vi "CRYDB Insert Into DatarunTable.vi"(6 "Station_ID":i32, 7 "Item_ID":i32, 8 "error in":errorcluster, 10 "Auto save":T1 {"Selector" items=["Space", "Underscores", "None"]}, 11 "connection reference":T2) -> (0 "error out":errorcluster, 2 "Datarun_ID":i32, 3 "connection reference out":T2)   [LabVIEW 2013]
uses:
  <vilib>/addons/database/Connection.llb/Conn ObjectReference.ctl
  Typedef Control/CRYAuto Save Cluster.ctl
  <vilib>/addons/database/Auxilliary.llb/DB Tools Column Info.ctl
  <vilib>/addons/database/Auxilliary.llb/DB Tools DataTypes.ctl
  Calibration/SubVI/CRYCal Global.vi
  CRYProject/CRYProject Editor Global.vi
  <vilib>/addons/database/Connection.llb/Conn Execute.vi
  <vilib>/addons/database/Recordset.llb/Rec Fetch Recordset Data (R).vi
  <vilib>/addons/database/Recordset.llb/Rec Destroy - Connection.vi
  <vilib>/addons/database/_DB Variant To Data/Database Variant To Data.xnode
  <vilib>/addons/database/NI_Database_API.lvlib
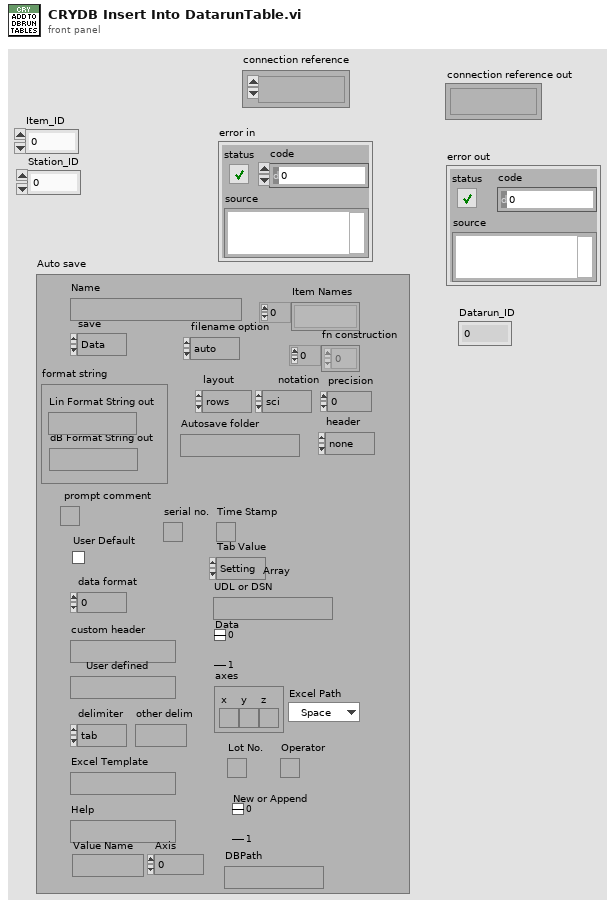
[diagram p1: front panel]
types:
  T1 = typedef "CRYAuto Save Cluster.ctl" = cluster{"Name":string, "save":enum16{"Data", "Results", "Waveforms"}, "Item Names":string[], "Autosave folder":path, "data format":u16, "filename option":enum16{"auto", "prompt"}, "fn construction":i32[], "layout":enum16{"rows", "columns"}, "notation":enum16{"sci", "float"}, "precision":i32, "prompt comment":bool, "header":enum16{"none", "standard", "custom"}, "custom header":string, "serial no.":bool, "User defined":string, "delimiter":enum16{"tab", "comma", "space", "other"}, "other delim":string, "axes":cluster{"x":bool, "y":bool, "z":bool}, "Time Stamp":bool, "Lot No.":bool, "Operator":bool, "Excel Template":string, "New or Append":u16, "Data":u16, "Help":string, "Tab Value":enum32{"Setting", "Help"}, "UDL or DSN":path, "User Default":bool, "Selector":i32, "Axis":u16, "Value Name":string, "format string":cluster{"dB Format String out":string, "Lin Format String out":string}, "DBPath":path}
  T2 = typedef "NI_Database_API.lvlib/Conn ObjectReference.ctl" = refnum<k1>
  T3 = typedef "NI_Database_API.lvlib/DB Tools Column Info.ctl" = cluster{"column name":string, "data type":T4, "size":i32, "allow null?":bool}
  T4 = typedef "NI_Database_API.lvlib/DB Tools DataTypes.ctl" = enum16{"String", "Long (I32)", "Single (SGL)", "Double (DBL)", "Date/Time", "Binary"}
  T5 = cluster{"Datarun_ID":u32, "Station_ID":i32, "Operator":string, "TStamp":string, "Item_ID":i32, "Comment":string, "Seq Name":string}
  T6 = typedef "CRYTS.ctl" = cluster{"No.TS":u16, "TS File Path":path, "TS Name":string, "EditStepName":string, "Steps":T7[], "New State":bool, "Change State":bool, "Flattened CurveLib Data":string, "Document Data":string, "EditStepNo":u16, "Operator Start File":string, "Sequence Type":string, "Sequence Language":string}
  T7 = typedef "CRYStep.ctl" = cluster{"No.VI":i32, "Category":string, "StepName":string, "Seq setup flattened":string, "Comment":string, "Steps config.":bool[], "Jump config":i32[], "Start":dbl, "Increment":dbl, "Name":string, "Unit":string, "Y data":u16, "Y prefix":string, "Y dB ref":dbl, "Y unit":string, "Repeat State Array":cluster{"Start":dbl, "Increment":dbl, "Count":i32, "Num":i32}[]}
  T8 = typedef "NI_Database_API.lvlib/Rec ObjectReference.ctl" = refnum<k1>
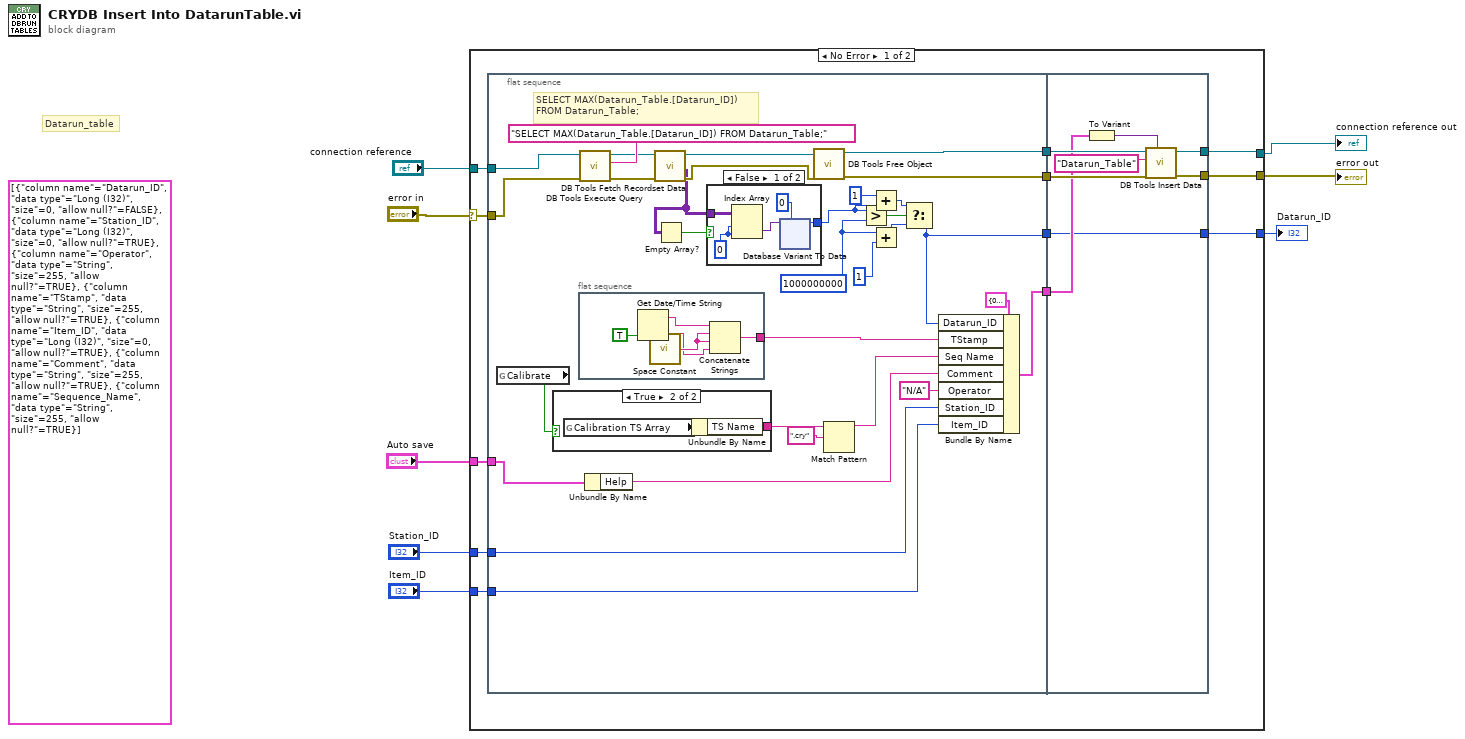
[diagram p0: block diagram]
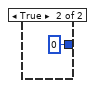
[diagram p2: hidden frame]
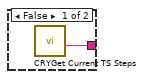
[diagram p3: hidden frame]
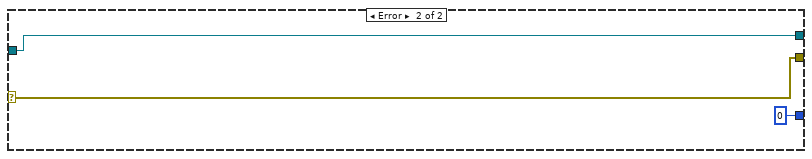
[diagram p4: hidden frame]
diagram:
  (unwired) T3[] [{"column name"="Datarun_ID", "data type"=enum."Long (I32)", "size"=0, "allow null?"=FALSE}, {"column name"="Station_ID", "data type"=enum."Long (I32)", "size"=0, "allow null?"=TRUE}, {"column name"="Operator", "data type"=enum."String", "size"=255, "allow null?"=TRUE}, {"column name"="TStamp", "data type"=enum."String", "size"=255, "allow null?"=TRUE}, {"column name"="Item_ID", "data type"=enum."Long (I32)", "size"=0, "allow null?"=TRUE}, {"column name"="Comment", "data type"=enum."String", "size"=255, "allow null?"=TRUE}, {"column name"="Sequence_Name", "data type"=enum."String", "size"=255, "allow null?"=TRUE}] ("column information")
  # "Datarun_table"
  n1 = case shown="No Error" "error in" {
    selector: "error in" -> [w17 w107]
    tunnel: "connection reference" -> [w20 w108]
    tunnel: [w15 w108] -> w5
    tunnel: [w14 w107] -> w6
    tunnel: "Auto save" -> [w13 _]
    tunnel: "Item_ID" -> [w12 _]
    tunnel: "Station_ID" -> [w11 _]
    tunnel: [w9 0] -> w1
    frame No Error {
      n2 = flat-sequence {
        tunnel: w20 -> [w51]
        tunnel: [w47] -> w19
        tunnel: [w40] -> w18
        tunnel: w17 -> [w39]
        tunnel: [w36] -> w16
        tunnel: w13 -> [w29]
        tunnel: w12 -> [w26]
        tunnel: w11 -> [w27]
        tunnel: [w24] -> w10
        tunnel: w19 -> [w105]
        tunnel: w18 -> [w99]
        tunnel: w16 -> [w103]
        tunnel: [w101] -> w15
        tunnel: [w100] -> w14
        tunnel: w10 -> [w98]
        tunnel: [w98] -> w9
        frame #0 {
          w43 = 1000000000 ("y")
          # "SELECT MAX(Datarun_Table.[Datarun_ID])\nFROM Datarun_Table;"
          n3 = global read "CRYCal Global.vi" "Calibrate"() -> (w34:bool)
          n4 = case shown="True" w34 {
            tunnel: [w95 w96] -> w32
            frame False {
              n5 = call "CRYGet Current TS Steps.vi"() -> ("TS Name"=w95:string)  [unwired: 7 in, 4 out]
            }
            frame True {
              n6 = global read "CRYProject Editor Global.vi" "Calibration TS Array"() -> (w97:T6)
              n7 = Unbundle By Name(w97) -> ("TS Name"=w96:string)
            }
          }
          n8 = flat-sequence {
            tunnel: [w90] -> w31
            frame #0 {
              n9 = Get Date/Time String(want seconds? (F)=TRUE) -> (date string=w94:string, time string=w91:string)  [unwired: 2 in]
              n10 = call <vilib>:"Space Constant.vi"() -> ("String"=w92:string)
              n11 = Concatenate Strings(w94, w92, w92, w91) -> (w90:string)
            }
          }
          n12 = call-poly <vilib>:"DB Tools Execute Query.vi"("error in (no error)"=w39, "SQL query"="SELECT MAX(Datarun_Table.[Datarun_ID]) FROM Datarun_Table;", "connection reference"=w51) -> ("error out"=w38:errorcluster, "recordset reference"=w49:T8)  [unwired: 5 in]
          n13 = Unbundle By Name(w29) -> ("Help"=w28:string)
          n14 = call-poly <vilib>:"DB Tools Fetch Recordset Data.vi"("error in (no error)"=w38, "recordset reference"=w49) -> ("error out"=w37:errorcluster, "recordset data"=w21:variant[][], "recordset reference out"=w48:T8)  [unwired: 3 in]
          n15 = Empty Array?(array=w21) -> (empty?=w23:bool)
          n16 = case shown="False" w23 {
            tunnel: w21 -> [w56 _]
            tunnel: [w53 0 ("data")] -> w22
            frame False {
              w55 = 0 ("disabled index (col)")
              n17 = Index Array(array=w56, index (row)=w55, index (col)=w55) -> (element=w52:variant)
              n18 = xnode "Database Variant To Data"("database variant"=w52, "type"=0) -> ("data"=w53:i32)  [unwired: 1 in, 1 out]
            }
            frame True {
            }
          }
          n19 = call-poly <vilib>:"DB Tools Free Object.vi"("error in (no error)"=w37, "recordset reference"=w48) -> ("error out"=w36:errorcluster, "connection reference"=w47:T2)  [unwired: 8 in]
          n20 = Match Pattern(string=w32, regular expression=".cry") -> (before substring=w30:string)  [unwired: 1 in, 3 out]
          n21 = Greater?(x=w22, y=w43) -> (0:w46:bool)
          n22 = Add(x=1, y=w22) -> (x+y=w41:i32)
          n23 = Add(x=w43, y=1 ("x")) -> (x+y=w44:i32)
          n24 = Select(t=w41, s=w46, f=w44) -> (s? t:f=w24:i32)
          n25 = Bundle By Name(cluster=T5 {"Datarun_ID"=0, "Station_ID"=0, "Operator"="", "TStamp"="", "Item_ID"=0, "Comment"="", "Seq Name"=""} ("DatarunTable Data"), "Datarun_ID"=w24, "TStamp"=w31, "Seq Name"=w30, "Comment"=w28, "Operator"="N/A", "Station_ID"=w27, "Item_ID"=w26) -> (w40:T5)
        }
        frame #1 {
          n26 = To Variant(anything=w99) -> (Variant=w102:variant)
          n27 = call <vilib>:"DB Tools Insert Data.vi"("data"=w102, "error in (no error)"=w103, "table"="Datarun_Table", "connection reference"=w105) -> ("error out"=w100:errorcluster, "connection reference out"=w101:T2)  [unwired: 6 in]
        }
      }
    }
    frame Error {
    }
  }
  "connection reference out" <- w5
  "error out" <- w6
  "Datarun_ID" <- w1
